vi "Has Next.vi"(8 "error in (no error)":errorcluster, 11 "UTF8 in":refnum<class "UTF-8 String.lvclass">) -> (0 "error out":errorcluster, 2 "Has Next?":bool, 3 "UTF8 out":refnum<class "UTF-8 String.lvclass">)   [LabVIEW 2010, in "JKI Unicode.lvlib" / "UTF-8 String.lvclass"]
uses:
  UTF-8 String.lvclass
  UTF-8 String.lvclass/UTF-8 String.ctl
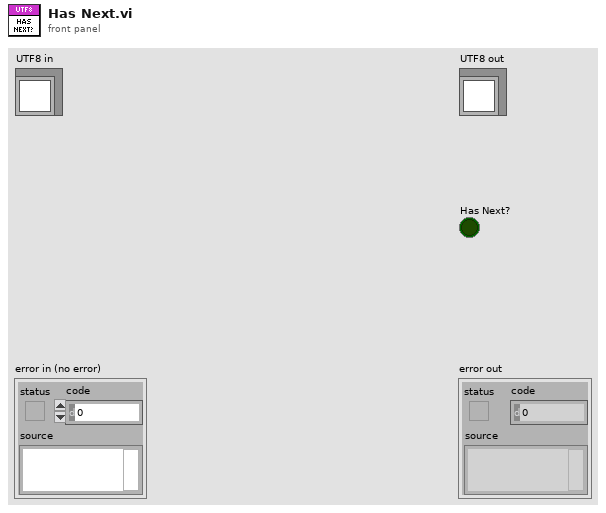
[diagram p1: front panel]
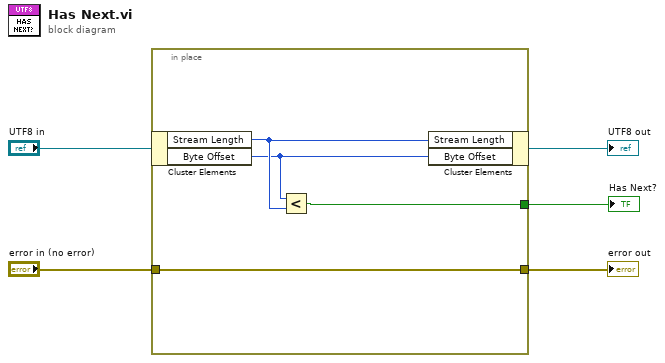
[diagram p0: block diagram]
diagram:
  n1 = in-place {
    in-place-border: "error in (no error)" -> [w7]
    in-place-border: [w8] -> w2
    in-place-border: [w7] -> w1
    n2 = in-place-cluster #1("UTF8 in") -> ("Stream Length"=w9:i32, "Byte Offset"=w6:i32)
    n3 = Less?(x=w6, y=w9) -> (x < y?=w8:bool)
    n4 = in-place-cluster #1("Stream Length"=w9, "Byte Offset"=w6) -> (→"UTF8 out":refnum<class "UTF-8 String.lvclass">)
  }
  "error out" <- w1
  "Has Next?" <- w2
